vi "display.vi"(8 "error in (no error)":errorcluster, 11 "ForecastDisplay in":refnum<class "ForecastDisplay.lvclass">) -> (0 "error out":errorcluster, 3 "ForecastDisplay out":refnum<class "ForecastDisplay.lvclass">)   [LabVIEW 2018, in "ForecastDisplay.lvclass"]
uses:
  ForecastDisplay.lvclass
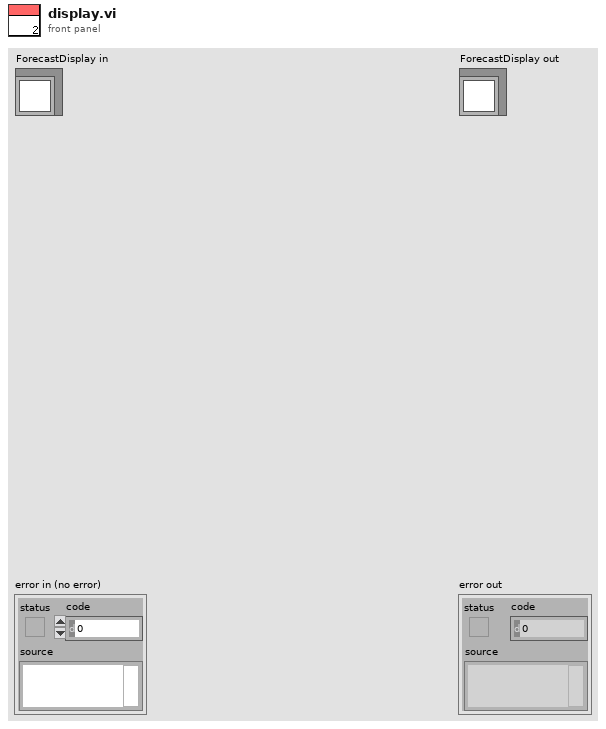
[diagram p1: front panel]
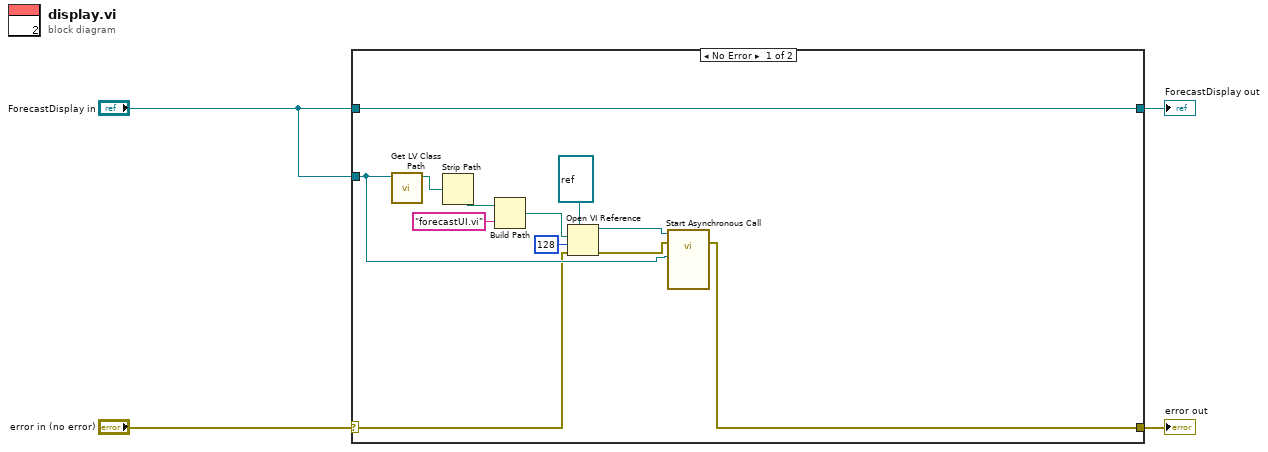
[diagram p0: block diagram]
diagram:
  n1 = case shown="No Error" "error in (no error)" {
    selector: "error in (no error)" -> [w6 w18]
    tunnel: [w5 w18] -> w3
    tunnel: [w16 w17] -> w2
    tunnel: "ForecastDisplay in" -> [w16 w17]
    tunnel: "ForecastDisplay in" -> [w9 _]
    frame No Error {
      n2 = call <vilib>:"Get LV Class Path.vi"("object"=w9) -> ("class path"=w15:path)  [unwired: 9 in, 1 out]
      n3 = Strip Path(path=w15) -> (stripped path=w7:path)  [unwired: 1 out]
      n4 = Build Path(base path=w7, name or relative path="forecastUI.vi") -> (appended path=w13:path)
      n5 = Open VI Reference(type specifier VI Refnum (for type only)=refnum<vi> refnum, vi path=w13, options=128, error in (no error)=w6) -> (vi reference=w11:refnum<vi>, error out=w10:errorcluster)  [unwired: 2 in]
      n6 = call-by-ref "Start Asynchronous Call"(reference=w11, error in=w10, "ForecastDisplay in"=w9) -> (error out=w5:errorcluster)  [unwired: 11 in, 1 out]
    }
    frame Error {
    }
  }
  "error out" <- w3
  "ForecastDisplay out" <- w2
